vi "Read Temperature DBL.vi"(8 "Error In":errorcluster, 10 "Source":string, 11 "reference in":refnum<class "Thermometer Multichannel.lvclass">) -> (0 "Error Out":errorcluster, 1 "Time Stamp":timestamp format="%<%x %.3X>T", 2 "Temperature":dbl, 3 "reference out":refnum<class "Thermometer Multichannel.lvclass">)   [LabVIEW 2024, in "Thermometer Multichannel.lvclass"]
uses:
  Thermometer Multichannel.lvclass
  Thermometer Multichannel Worker/Thermometer Multichannel Worker Messages/Get Temperature DBL Msg/Get Temperature DBL Msg.lvclass/Get Temperature DBL Msg.ctl
  <vilib>/ActorFramework/Reply Msg/Reply Msg.lvclass/Reply Msg.ctl
  <vilib>/ActorFramework/Message Enqueuer/Message Enqueuer.lvclass/Message Enqueuer.ctl
  Thermometer Multichannel Worker/Thermometer Multichannel Worker Messages/Get Temperature DBL Msg/Get Temperature DBL Msg.lvclass
  C:/Program Files/National Instruments/LabVIEW 2025/vi.lib/ActorFramework/Reply Msg/Reply Msg.lvclass
  <vilib>/ActorFramework/Reply Msg/Reply Msg.lvclass
  C:/Program Files/National Instruments/LabVIEW 2025/vi.lib/ActorFramework/Message/Message.lvclass
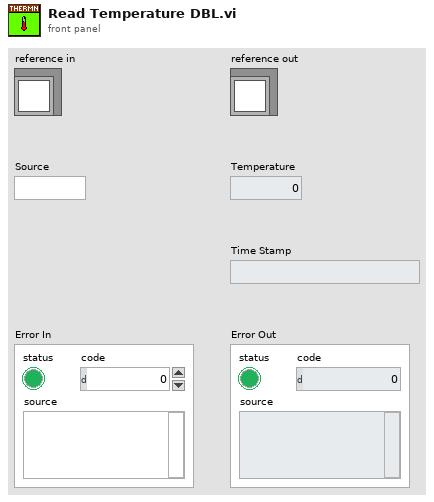
[diagram p1: front panel]
types:
  T1 = typedef "Thermometer Multichannel.lvclass/ObjectAttributes.ctl" = cluster{"IConfigure":refnum<class "IConfigure.lvclass">, "Worker Enqueuer":refnum<class "Message Enqueuer.lvclass">}
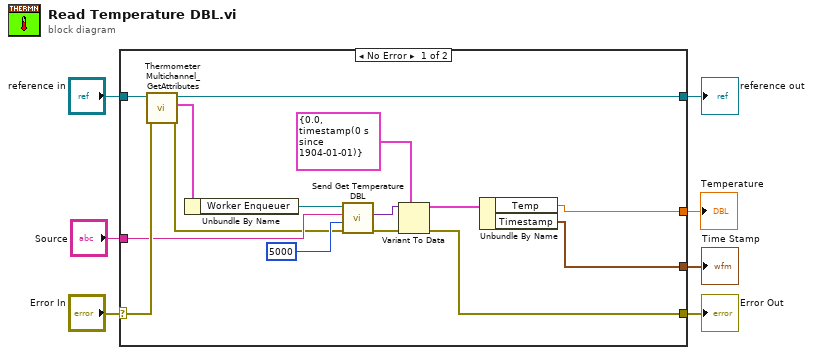
[diagram p0: block diagram]
diagram:
  n1 = case shown="No Error" "Error In" {
    selector: "Error In" -> [w22 w24]
    tunnel: [w13 w24] -> w6
    tunnel: [w19 w23] -> w4
    tunnel: "reference in" -> [w20 w23]
    tunnel: "Source" -> [w17 _]
    tunnel: [w8 _] -> w2
    tunnel: [w9 _] -> w1
    frame No Error {
      n2 = call "Thermometer Multichannel_GetAttributes.vi"("Error In"=w22, "reference in"=w20) -> ("Error Out"=w15:errorcluster, "Data"=w21:T1, "reference out"=w19:refnum<class "Thermometer Multichannel.lvclass">)  [unwired: 6 in, 1 out]
      n3 = Unbundle By Name(w21) -> ("Worker Enqueuer"=w18:refnum<class "Message Enqueuer.lvclass">)
      n4 = call "Send Get Temperature DBL.vi"("error in (no error)"=w15, "timeout in ms (-1)"=5000, "Source"=w17, "Message Enqueuer"=w18) -> ("error out"=w14:errorcluster, "Reply"=w12:variant)  [unwired: 4 in, 2 out]
      n5 = Variant To Data(error in=w14, type=cluster{"Temp":dbl, "Timestamp":timestamp} {"Temp"=0.0, "Timestamp"=timestamp(0 s since 1904-01-01)}, Variant=w12) -> (data=w10:cluster{"Temp":dbl, "Timestamp":timestamp}, error out=w13:errorcluster)
      n6 = Unbundle By Name(w10) -> ("Temp"=w8:dbl, "Timestamp"=w9:timestamp)
    }
    frame Error {
    }
  }
  "Error Out" <- w6
  "reference out" <- w4
  "Time Stamp" <- w1
  "Temperature" <- w2
